vi "to string.vi"(8 "error in":errorcluster, 11 "channel in":refnum<class "EIP Tags Channel.lvclass">) -> (0 "error out":errorcluster, 1 "channel data":string, 2 "identifier":string, 3 "channel out":refnum<class "EIP Tags Channel.lvclass">)   [LabVIEW 2013, in "EIP Tags Channel.lvclass"]
doc: "NI Tag Bus Module Framework 1.0.3.46\nNI Systems Engineering"
uses:
  EIP Tags Channel.lvclass
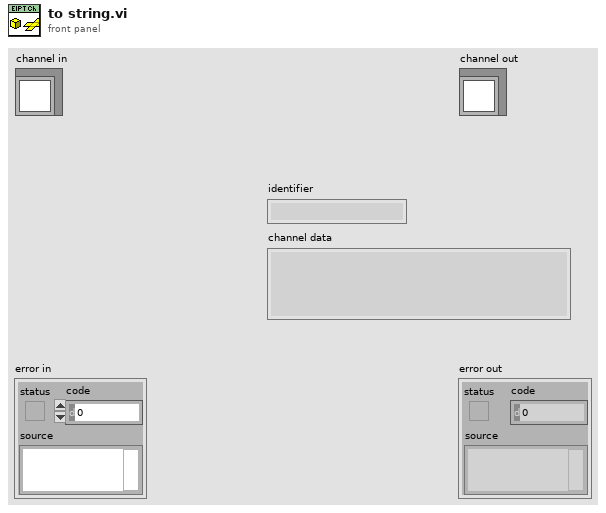
[diagram p1: front panel]
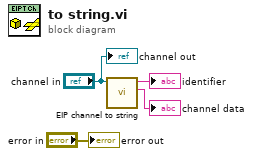
[diagram p0: block diagram]
diagram:
  n1 = call "EIP channel to string.vi"("channel in"="channel in") -> ("channel data"=→"channel data":string, "identifier"=→"identifier":string)  [unwired: 9 in]
  "error out" <- "error in"
  "channel out" <- "channel in"
